vi "residues of one root.vi"(8 "index of root":i32, 9 "multiplicity of roots":i32[](array[numeric]), 10 "roots":cdb[](array[numeric]) format="%#.2g", 11 "Rest":cdb[](array[numeric]) format="%#.2g") -> (3 "Residues of root":cdb[](array[numeric]))   [LabVIEW 2020, in "NI_AALPro.lvlib"]
uses:
  NI_AALPro.lvlib
  Add Polynomials (CDB).vi
  Multiply Polynomials (CDB).vi
  Subtract Polynomials (CDB).vi
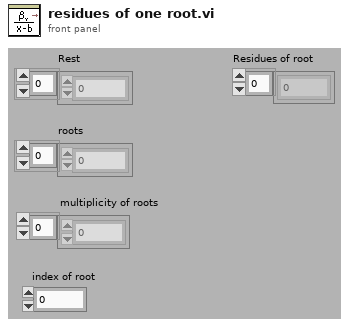
[diagram p1: front panel]
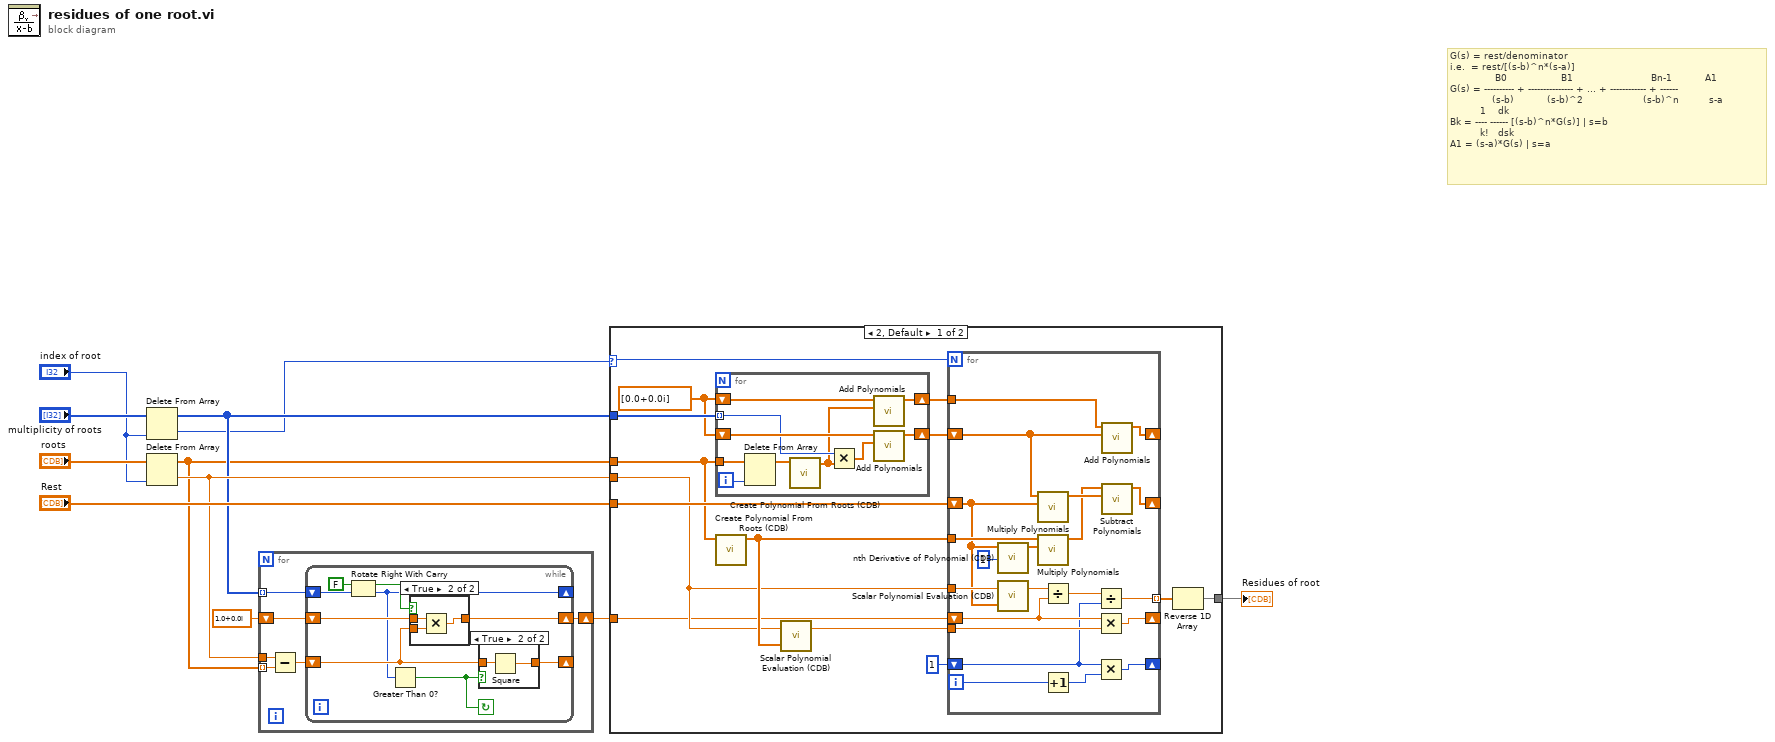
[diagram p0: block diagram]
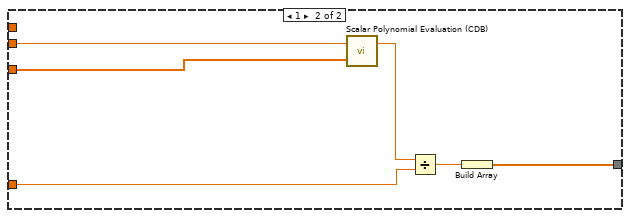
[diagram p4: hidden frame]
diagram:
  # "G(s) = rest/denominator   \ni.e.  = rest/[(s-b)^n*(s-a)]\n               B0                  B1                          Bn-1           A1\nG(s) = ---------- + --------------- + ... + ------------ + ------\n              (s-b)           (s-b)^2                    (s-b)^n          s-a\n          1    dk\nBk = ---- ------ [(s-b)^n*G(s)] | s=b \n          k!   dsk\nA1 = (s-a)*G(s) | s=a"
  n1 = Delete From Array(array="multiplicity of roots", index="index of root") -> (deleted portion=w2:i32, array with subset deleted=w4:i32[])  [unwired: 1 in]
  n2 = Delete From Array(array="roots", index="index of root") -> (deleted portion=w6:cdb, array with subset deleted=w1:cdb[])  [unwired: 1 in]
  n3 = for {
    tunnel: w1 -> [w16] mode=indexing
    tunnel: w4 -> [w13] mode=indexing
    shift-right: [w14] -> w8
    shift-left: cdb 1.0+0.0i -> [w15]
    tunnel: w6 -> [w17]
    n4 = Subtract(x=w17, y=w16) -> (x-y=w12:cdb)
    n5 = while {
      shift-right: [w21] -> w14
      shift-left: w15 -> [w22]
      shift-right: [w26] -> _
      shift-left: w12 -> [w20]
      shift-right: [w19] -> _
      shift-left: w13 -> [w25]
      stop <- w18 continue-if-true
      n6 = Rotate Right With Carry(2:w25, 3:FALSE ("carry")) -> (0:w19:i32, 1:w23:bool)
      n7 = Greater Than 0?(x=w19) -> (x > 0?=w18:bool)
      n8 = case shown="True" w23 {
        tunnel: w22 -> [w30 w32]
        tunnel: [w30 w33] -> w21
        tunnel: w20 -> [_ w31]
        frame False {
        }
        frame True {
          n9 = Multiply(x=w32, y=w31) -> (x*y=w33:cdb)
        }
      }
      n10 = case shown="True" w18 {
        tunnel: [w27 w29] -> w26
        tunnel: w20 -> [w27 w28]
        frame False {
        }
        frame True {
          n11 = Square(x=w28) -> (x^2=w29:cdb)
        }
      }
    }
  }
  n12 = case shown="2, Default" w2 {
    selector: w2 -> [w43 _]
    tunnel: "Rest" -> [w46 w84]
    tunnel: [w47 w81] -> w10
    tunnel: w6 -> [w42 w80]
    tunnel: w8 -> [w41 w79]
    tunnel: w4 -> [w37 _]
    tunnel: w1 -> [w38 _]
    frame 2, Default {
      w34 = cdb[] [0.0+0.0i] ("P(x)+Q(x)")
      n13 = for {
        tunnel: w38 -> [w57]
        tunnel: w37 -> [w51] mode=indexing
        shift-right: [w54] -> w36
        shift-left: w34 -> [w52]
        shift-right: [w50] -> w35
        shift-left: w34 -> [w49]
        i -> [w56]
        n14 = Delete From Array(array=w57, index=w56) -> (array with subset deleted=w55:cdb[])  [unwired: 1 in, 1 out]
        n15 = call "Create Polynomial From Roots (CDB).vi"("Roots"=w55) -> ("P(x)"=w48:cdb[])  [unwired: 9 in, 1 out]
        n16 = Multiply(x=w51, y=w48) -> (x*y=w53:cdb[])
        n17 = call-poly "Add Polynomials.vi"("Q(x)"=w48, "P(x)"=w49) -> ("P(x)+Q(x)"=w50:cdb[])  [unwired: 8 in, 1 out]
        n18 = call-poly "Add Polynomials.vi"("Q(x)"=w53, "P(x)"=w52) -> ("P(x)+Q(x)"=w54:cdb[])  [unwired: 8 in, 1 out]
      }
      n19 = call "Create Polynomial From Roots (CDB).vi"("Roots"=w38) -> ("P(x)"=w45:cdb[])  [unwired: 9 in, 1 out]
      n20 = call "Scalar Polynomial Evaluation (CDB).vi"("P(x)"=w45, "a"=w42) -> ("P(a)"=w40:cdb)  [unwired: 1 out]
      n21 = for {
        N: w43 -> [_]
        shift-right: [w75] -> _
        shift-left: w46 -> [w63]
        tunnel: w45 -> [w76]
        shift-right: [w66] -> _
        shift-left: w41 -> [w67]
        shift-right: [w65] -> _
        shift-left: 1 -> [w64]
        tunnel: [w71] -> w44 mode=indexing
        tunnel: w42 -> [w70]
        tunnel: w40 -> [w69]
        tunnel: w35 -> [w59]
        shift-right: [w60] -> _
        shift-left: w36 -> [w58]
        i -> [w74]
        n22 = call "nth Derivative of Polynomial (CDB).vi"("order"=1, "P(x)"=w63) -> ("Nth Derivative of P(x)"=w77:cdb[])  [unwired: 8 in, 1 out]
        n23 = call "Scalar Polynomial Evaluation (CDB).vi"("P(x)"=w63, "a"=w70) -> ("P(a)"=w73:cdb)  [unwired: 1 out]
        n24 = call-poly "Multiply Polynomials.vi"("Q(x)"=w63, "P(x)"=w58) -> ("P(x)*Q(x)"=w62:cdb[])  [unwired: 8 in, 1 out]
        n25 = call-poly "Multiply Polynomials.vi"("Q(x)"=w77, "P(x)"=w76) -> ("P(x)*Q(x)"=w61:cdb[])  [unwired: 8 in, 1 out]
        n26 = Divide(x=w73, y=w67) -> (x/y=w72:cdb)
        n27 = Increment(x=w74) -> (x+1=w68:i32)
        n28 = Divide(x=w72, y=w64) -> (x/y=w71:cdb)
        n29 = Multiply(x=w67, y=w69) -> (x*y=w66:cdb)
        n30 = Multiply(x=w64, y=w68) -> (x*y=w65:i32)
        n31 = call-poly "Add Polynomials.vi"("Q(x)"=w58, "P(x)"=w59) -> ("P(x)+Q(x)"=w60:cdb[])  [unwired: 8 in, 1 out]
        n32 = call-poly "Subtract Polynomials.vi"("Q(x)"=w62, "P(x)"=w61) -> ("P(x)-Q(x)"=w75:cdb[])  [unwired: 8 in, 1 out]
      }
      n33 = Reverse 1D Array(array=w44) -> (reversed array=w47:cdb[])
    }
    frame 1 {
      n34 = call "Scalar Polynomial Evaluation (CDB).vi"("P(x)"=w84, "a"=w80) -> ("P(a)"=w83:cdb)  [unwired: 1 out]
      n35 = Divide(x=w83, y=w79) -> (x/y=w82:cdb)
      n36 = Build Array(w82) -> (w81:cdb[])
    }
  }
  "Residues of root" <- w10
